vi "Delete Array Element.vi"(5 "Key name":string, 6 "Index":i32=4, 7 "Section name":string, 8 "error in (no error)":errorcluster, 9 "Use Key Regex? [F]":bool, 10 "Use Section Regex? [F]":bool, 11 "Carya Config in":refnum<class "Carya Config.lvclass">) -> (0 "error out":errorcluster, 3 "Carya Config out":refnum<class "Carya Config.lvclass">)   [LabVIEW 2013, in "Carya Config.lvclass"]
doc: "Copyright 2018, Carya Automatisering, Wiebe Walstra."
uses:
  Carya Config.lvclass
  CConfig Object/Search Replace Query/Search Replace Query.lvclass
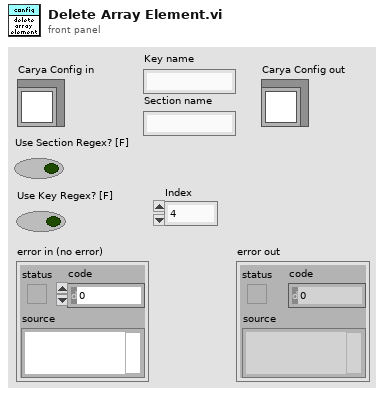
[diagram p1: front panel]
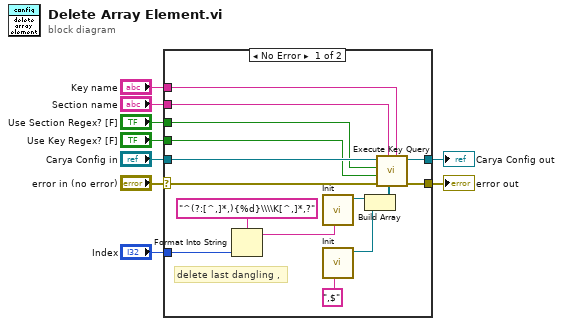
[diagram p0: block diagram]
diagram:
  n1 = case shown="No Error" "error in (no error)" {
    selector: "error in (no error)" -> [w24 w26]
    tunnel: [w23 w26] -> w8
    tunnel: [w22 w25] -> w6
    tunnel: "Carya Config in" -> [w21 w25]
    tunnel: "Section name" -> [w18 _]
    tunnel: "Key name" -> [w17 _]
    tunnel: "Use Section Regex? [F]" -> [w20 _]
    tunnel: "Use Key Regex? [F]" -> [w19 _]
    tunnel: "Index" -> [w14 _]
    frame No Error {
      # "delete last dangling ,"
      n2 = Format Into String(format string="^(?:[^,]*,){%d}\\\\K[^,]*,?" ("Regex"), w14) -> (resulting string=w13:string)  [unwired: 2 in, 1 out]
      n3 = call "Init.vi"("Search"=w13) -> ("Find First Query out"=w16:refnum<class "Search Replace Query.lvclass">)  [unwired: 9 in, 1 out]
      n4 = call "Init.vi"("Search"=",$") -> ("Find First Query out"=w11:refnum<class "Search Replace Query.lvclass">)  [unwired: 9 in, 1 out]
      n5 = Build Array(w16, w11) -> (w15:refnum<class "Search Replace Query.lvclass">[])
      n6 = call-dynamic "Execute Key Query.vi"("Key name"=w17, "Key queries"=w15, "Section name"=w18, "error in (no error)"=w24, "Use Key Regex? [F]"=w19, "Use Section Regex? [F]"=w20, "Carya Config in"=w21) -> ("error out"=w23:errorcluster, "Carya Config out"=w22:refnum<class "Carya Config.lvclass">)  [unwired: 2 in, 1 out]
    }
    frame Error {
    }
  }
  "error out" <- w8
  "Carya Config out" <- w6
